vi "复制文本-选中累积剂量.vi"(11 "引用-数据列表":refnum<vi>) -> (0 "错误输出":errorcluster, 2 "文本":string)   [LabVIEW 2017]
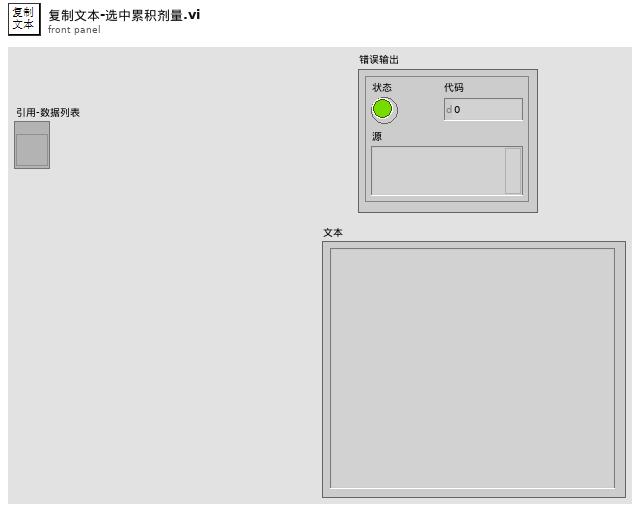
[diagram p1: front panel]
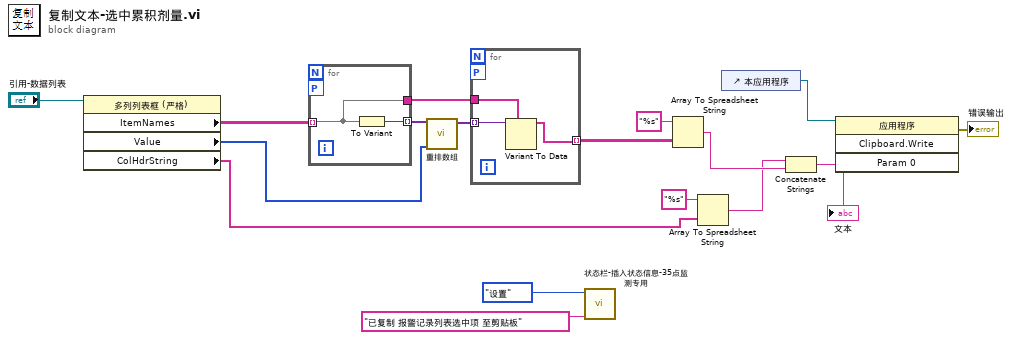
[diagram p0: block diagram]
diagram:
  n1 = property class="多列列表框 (严格)"(reference="引用-数据列表") -> ("ItemNames"=w5:string[][], "Value"=w4:i32[], "ColHdrString"=w3:string[])  [unwired: 1 in, 2 out]
  n2 = for {
    tunnel: w5 -> [w18] mode=indexing
    tunnel: [w19] -> w17 mode=indexing
    tunnel: [w18] -> w15
    workers-P: _ -> [_]
    n3 = To Variant(anything=w18) -> (Variant=w19:variant)
  }
  n4 = call "重排数组.vi"("新索引顺序"=w4, "原数组"=w17) -> ("排序后数组"=w16:variant[])  [unwired: 9 in]
  n5 = for {
    tunnel: w16 -> [w22] mode=indexing
    tunnel: w15 -> [w21]
    tunnel: [w20] -> w14 mode=indexing
    workers-P: _ -> [_]
    n6 = Variant To Data(type=w21, Variant=w22) -> (data=w20:string[])  [unwired: 1 in, 1 out]
  }
  n7 = call "状态栏-插入状态信息-35点监测专用.vi"("消息内容"="已复制 报警记录列表选中项 至剪贴板", "状态类型"=enum16{"全部", "报警", "通信", "设置"}."设置") -> ()  [unwired: 10 in]
  n8 = Array To Spreadsheet String(array=w14, 3:"%s" ("格式字符串")) -> (spreadsheet string=w8:string)  [unwired: 1 in]
  n9 = Array To Spreadsheet String(array=w3, 3:"%s" ("格式字符串")) -> (spreadsheet string=w6:string)  [unwired: 1 in]
  n10 = control-ref of="本应用程序"() -> (w12:refnum<vi>)
  n11 = Concatenate Strings(w6, w8) -> (w7:string)
  "文本" <- w7
  n12 = invoke class="应用程序" method="Clipboard.Write"(reference=w12, "Param 0"=w7) -> (error out=→"错误输出":errorcluster)  [unwired: 2 in, 3 out]
